vi "MTMount_getSample_MirrorCoverLocks.vi"(8 "error in (no error)":errorcluster, 11 "Mirror_Cover_Locks_Ctl":T1) -> (0 "error out":errorcluster, 2 "function return":i32, 3 "Mirror_Cover_Locks_Ctl out":T1)   [LabVIEW 2018, in "SALLV_MTMount.lvlib"]
doc: "int MTMount_shm_getSample_Mirror_Cover_LocksLV(MTMount_Mirror_Cover_LocksLV *Mirror_Cover_Locks_Ctl );"
uses:
  SALLV_MTMount.lvlib
  DataTypes/Mirror_Cover_Locks.ctl
  SALLV_MTMount.so
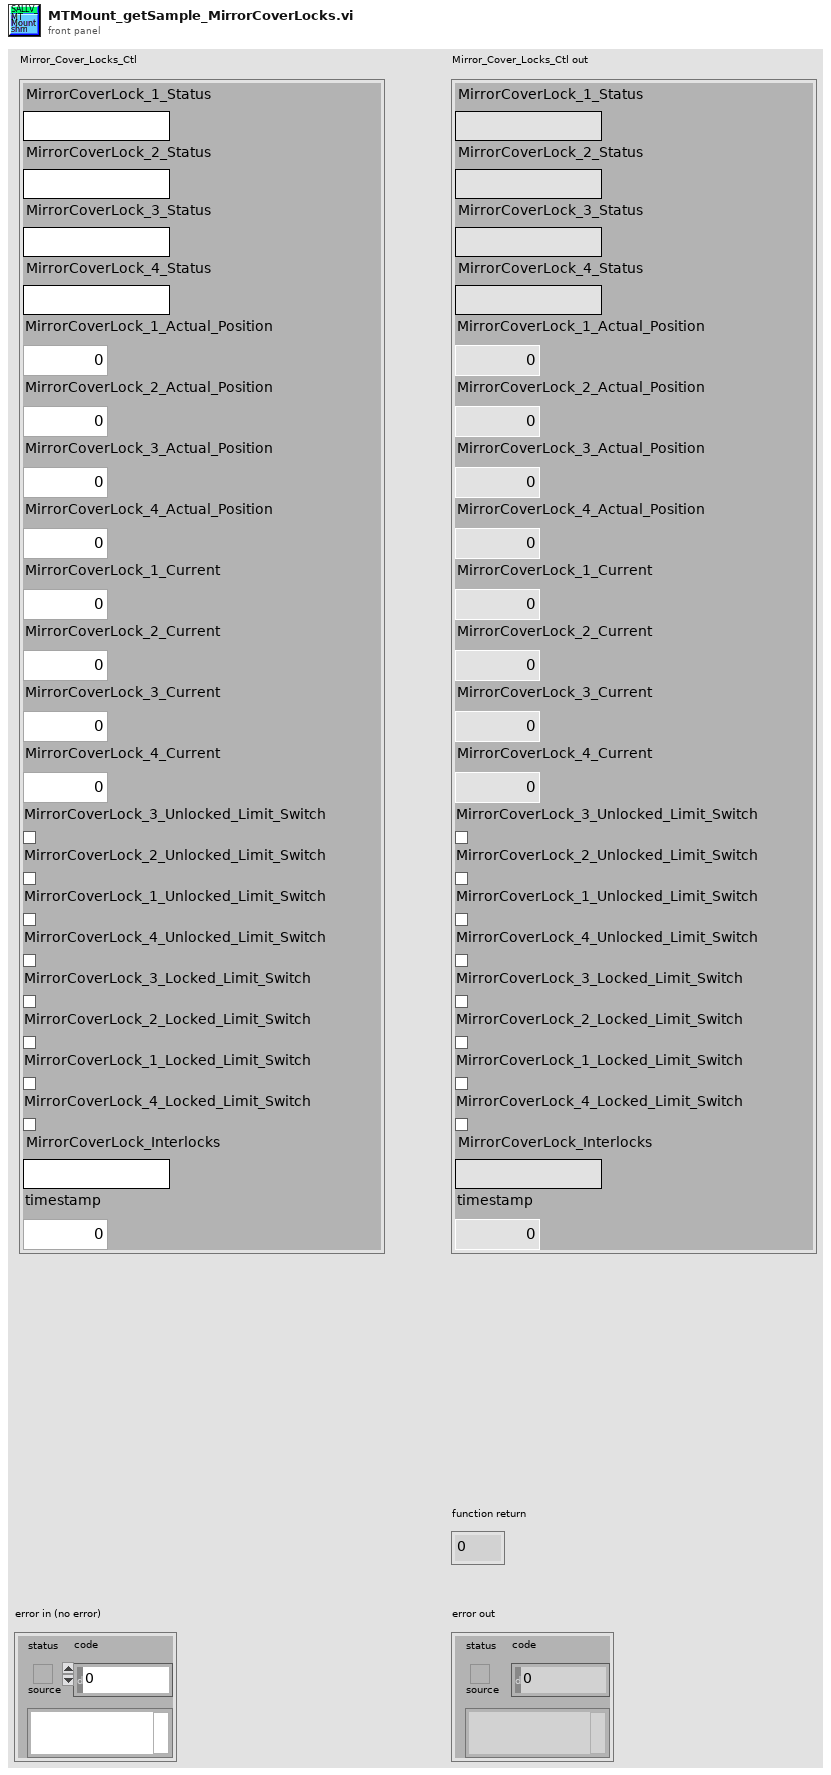
[diagram p1: front panel]
types:
  T1 = typedef "SALLV_MTMount.lvlib/Mirror_Cover_Locks.ctl" = cluster{"MirrorCoverLock_1_Status":string, "MirrorCoverLock_2_Status":string, "MirrorCoverLock_3_Status":string, "MirrorCoverLock_4_Status":string, "MirrorCoverLock_1_Actual_Position":dbl, "MirrorCoverLock_2_Actual_Position":dbl, "MirrorCoverLock_3_Actual_Position":dbl, "MirrorCoverLock_4_Actual_Position":dbl, "MirrorCoverLock_1_Current":dbl, "MirrorCoverLock_2_Current":dbl, "MirrorCoverLock_3_Current":dbl, "MirrorCoverLock_4_Current":dbl, "MirrorCoverLock_3_Unlocked_Limit_Switch":bool, "MirrorCoverLock_2_Unlocked_Limit_Switch":bool, "MirrorCoverLock_1_Unlocked_Limit_Switch":bool, "MirrorCoverLock_4_Unlocked_Limit_Switch":bool, "MirrorCoverLock_3_Locked_Limit_Switch":bool, "MirrorCoverLock_2_Locked_Limit_Switch":bool, "MirrorCoverLock_1_Locked_Limit_Switch":bool, "MirrorCoverLock_4_Locked_Limit_Switch":bool, "MirrorCoverLock_Interlocks":string, "timestamp":dbl}
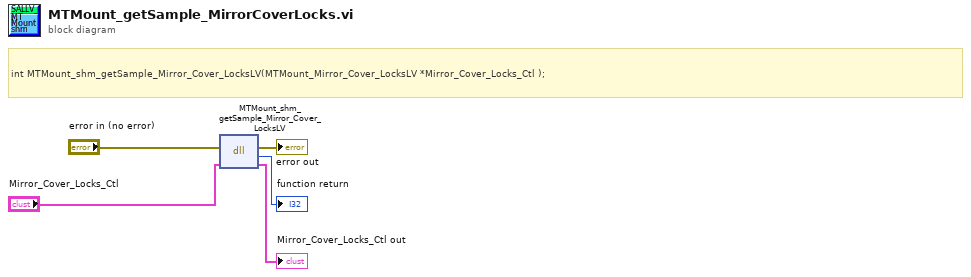
[diagram p0: block diagram]
diagram:
  # "int MTMount_shm_getSample_Mirror_Cover_LocksLV(MTMount_Mirror_Cover_LocksLV *Mirror_Cover_Locks_Ctl );"
  n1 = dll-call lib="home/ttsai/Document/salApiMTMount/SALLV_MTMount/SALLV_MTMount.*" fn="MTMount_shm_getSample_Mirror_Cover_LocksLV"(error in="error in (no error)", "Mirror_Cover_Locks_Ctl"="Mirror_Cover_Locks_Ctl") -> (error out=→"error out":errorcluster, →"function return":i32, "Mirror_Cover_Locks_Ctl"=→"Mirror_Cover_Locks_Ctl out":T1)  [unwired: 2 in, 1 out]
